vi "Save Enable ACQ.vi"(8 "error in (no error)":errorcluster, 10 "Save Enable":bool, 11 "ACQ Contador in":refnum<class "ACQ Contador.lvclass">) -> (0 "error out":errorcluster, 3 "ACQ Contador out":refnum<class "ACQ Contador.lvclass">)   [LabVIEW 2020, in "ACQ Contador.lvlib" / "ACQ Contador.lvclass"]
uses:
  ACQ Contador.lvclass
  ACQ Contador.lvclass/ACQ Contador.ctl
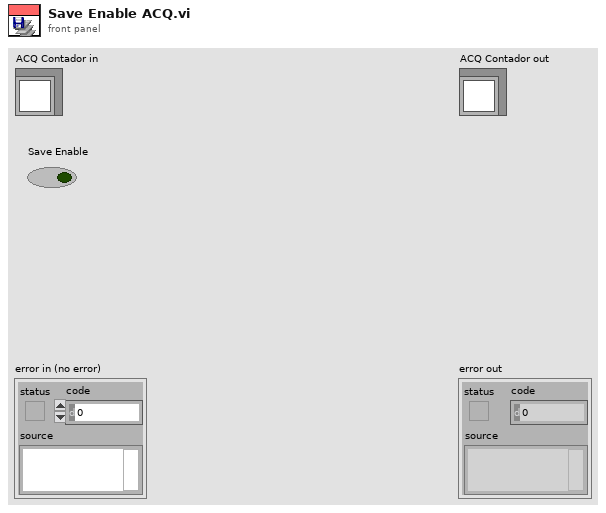
[diagram p1: front panel]
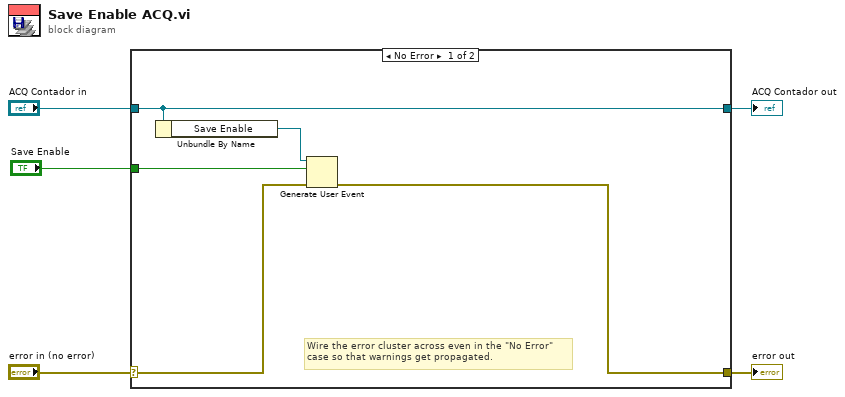
[diagram p0: block diagram]
diagram:
  n1 = case shown="No Error" "error in (no error)" {
    selector: "error in (no error)" -> [w7 w12]
    tunnel: [w6 w12] -> w4
    tunnel: [w10 w11] -> w2
    tunnel: "ACQ Contador in" -> [w10 w11]
    tunnel: "Save Enable" -> [w9 _]
    frame No Error {
      # "Wire the error cluster across even in the \"No Error\"\ncase so that warnings get propagated."
      n2 = Unbundle By Name(w10) -> ("Save Enable"=w8:refnum<user-event>)
      n3 = Generate User Event(user event=w8, event data cluster=w9, error in=w7) -> (error out=w6:errorcluster)  [unwired: 1 in, 1 out]
    }
    frame Error {
    }
  }
  "error out" <- w4
  "ACQ Contador out" <- w2
